vi "Set Correction on-off.vi"(8 "error in (no error)":errorcluster, 9 "interpolation/freq subset":bool=TRUE, 10 "correction":bool=TRUE, 11 "VISA resource name":refnum<visa-resource-name>) -> (0 "error out":errorcluster, 3 "VISA resource name out":refnum<visa-resource-name>)   [LabVIEW 2018, in "Agilent 87XX Series.lvlib"]
doc: "This VI for the HP8753B Network Analyzer and is used to turn correction and interpolation on and off."
uses:
  Agilent 87XX Series.lvlib
panel:
  # "ON\nOFF"
  # "ON\nOFF"
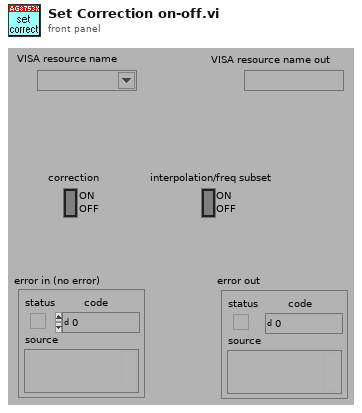
[diagram p1: front panel]
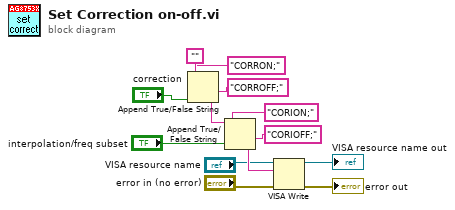
[diagram p0: block diagram]
diagram:
  n1 = Append True/False String(1:"correction", 2:"CORROFF;", 3:"CORRON;", 4:"") -> (0:w5:string)
  n2 = Append True/False String(1:"interpolation/freq subset", 2:"CORIOFF;", 3:"CORION;", 4:w5) -> (0:w3:string)
  n3 = VISA Write(VISA resource name="VISA resource name", write buffer=w3, error in (no error)="error in (no error)") -> (VISA resource name out=→"VISA resource name out":refnum<visa-resource-name>, error out=→"error out":errorcluster)  [unwired: 1 out]
